vi "read_delta.vi"(10 "Abort Delta":bool, 11 "Keithley":refnum<visa-resource-name>) -> (2 "aborted?":bool, 3 "delta reading [ohm]":dbl)   [LabVIEW 2019]
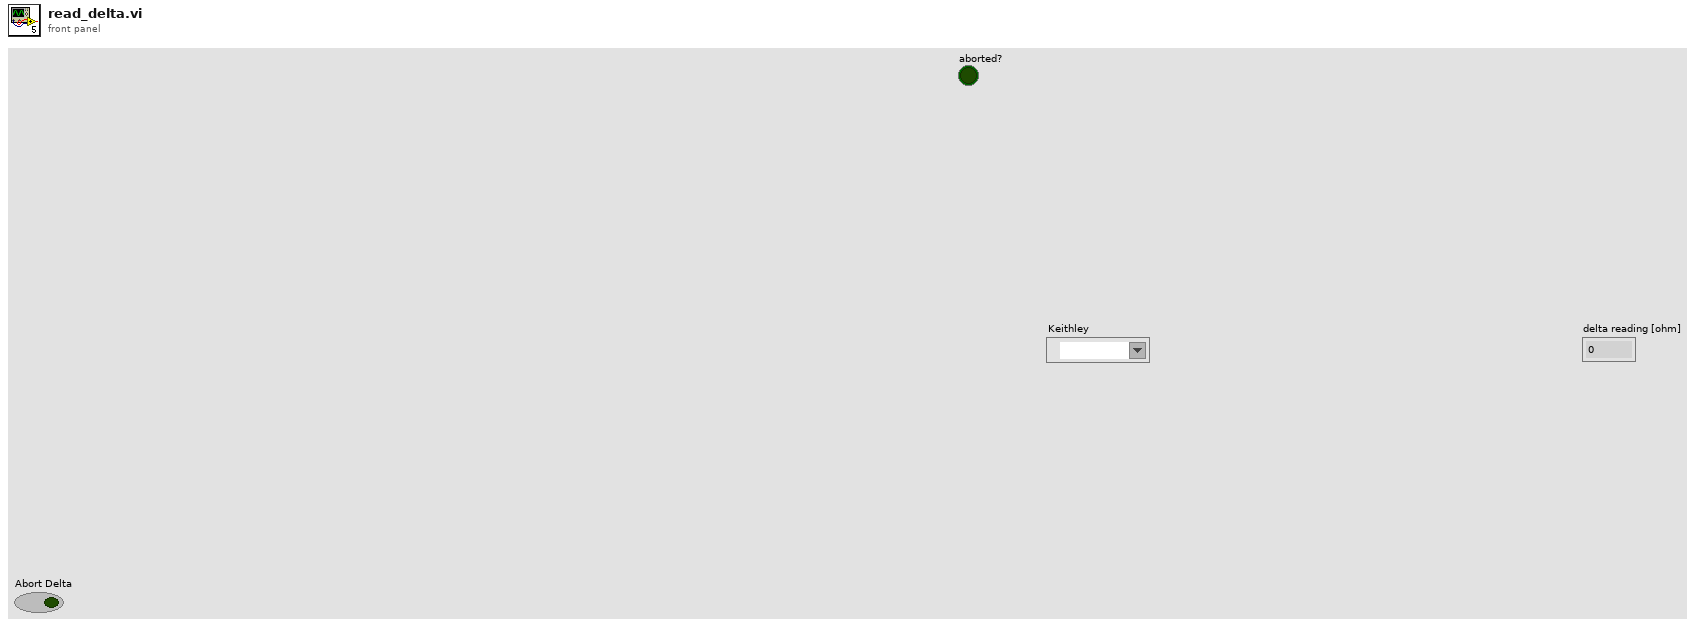
[diagram p1: front panel]
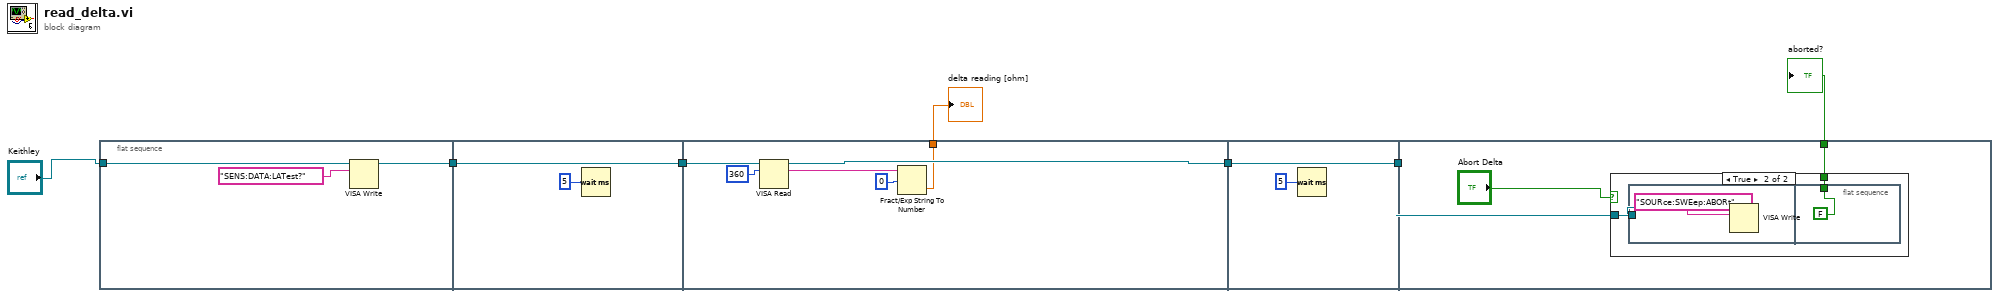
[diagram p0: block diagram]
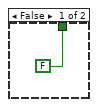
[diagram p2: hidden frame]
diagram:
  n1 = flat-sequence {
    tunnel: "Keithley" -> [w10]
    tunnel: [w8] -> w7
    tunnel: [w11] -> w6
    tunnel: w7 -> [w11]
    tunnel: w6 -> [w15]
    tunnel: [w14] -> w5
    tunnel: [w13] -> w3
    tunnel: [w19] -> w4
    tunnel: w5 -> [w19]
    tunnel: w4 -> [w22]
    tunnel: [w21] -> w1
    frame #0 {
      n2 = VISA Write(VISA resource name=w10, write buffer="SENS:DATA:LATest?" ("write buffer 2")) -> (VISA resource name out=w8:refnum<visa-resource-name>)  [unwired: 1 in, 2 out]
    }
    frame #1 {
      n3 = Wait (ms)(milliseconds to wait=5) -> ()  [unwired: 1 out]
    }
    frame #2 {
      n4 = VISA Read(VISA resource name=w15, byte count=u32 360) -> (VISA resource name out=w14:refnum<visa-resource-name>, read buffer=w17:string)  [unwired: 1 in, 2 out]
      n5 = Fract/Exp String To Number(string=w17, offset=0) -> (number=w13:dbl)  [unwired: 3 out]
    }
    frame #3 {
      n6 = Wait (ms)(milliseconds to wait=5) -> ()  [unwired: 1 out]
    }
    frame #4 {
      n7 = case shown="True" "Abort Delta" {
        tunnel: w22 -> [_ w26]
        tunnel: [FALSE w25] -> w21
        frame False {
        }
        frame True {
          n8 = flat-sequence {
            tunnel: w26 -> [w28]
            tunnel: [FALSE] -> w25
            frame #0 {
              n9 = VISA Write(VISA resource name=w28, write buffer="SOURce:SWEep:ABORt") -> ()  [unwired: 1 in, 3 out]
            }
            frame #1 {
            }
          }
        }
      }
    }
  }
  "delta reading [ohm]" <- w3
  "aborted?" <- w1
